vi "sendToRecycleBin.vi"(8 "error in":errorcluster, 11 "Directory to Recycle":path) -> (0 "error out":errorcluster)   [LabVIEW 2013, in "Project Wizard.lvlib"]
uses:
  Project Wizard.lvlib
  Microsoft.VisualBasic
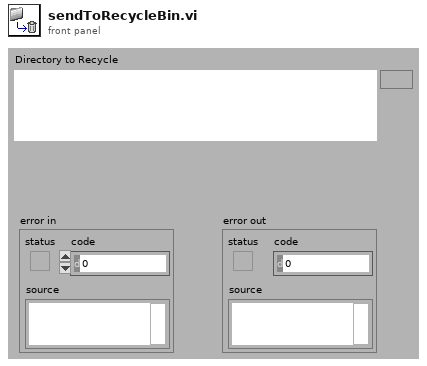
[diagram p1: front panel]
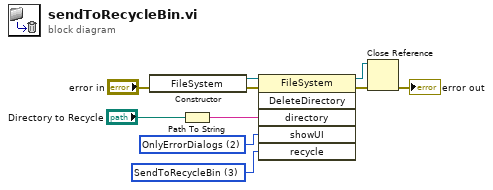
[diagram p0: block diagram]
diagram:
  w1 = 3 items=["DeletePermanently"=2, "SendToRecycleBin"=3] ("Delete Options (recycl")
  w2 = 2 items=["OnlyErrorDialogs"=2, "AllDialogs"=3] ("Dialog Options (only errors)")
  n1 = constructor class="FileSystem"(error in="error in") -> (reference out=w9:refnum<k24>, error out=w10:errorcluster)  [unwired: 2 in, 1 out]
  n2 = Path To String(path="Directory to Recycle") -> (string=w3:string)
  n3 = invoke class="FileSystem" method="DeleteDirectory"(reference=w9, error in=w10, "directory"=w3, "showUI"=w2, "recycle"=w1) -> (reference out=w7:refnum<k24>, error out=w6:errorcluster)  [unwired: 1 in, 4 out]
  n4 = Close Reference(reference=w7, error in (no error)=w6) -> (error out=→"error out":errorcluster)
